vi "Write configuration.vi"(8 "error in (no error)":errorcluster, 11 "Template in":refnum<class "Cobolt.lvclass">=refnum) -> (0 "error out":errorcluster, 3 "Template out":refnum<class "Cobolt.lvclass">)   [LabVIEW 2012, in "Cobolt.lvclass"]
doc: "Writes the configuration cluster into the configuration file. Configuration file is XML-based. It's name is <component ID>.xml"
uses:
  Cobolt.lvclass
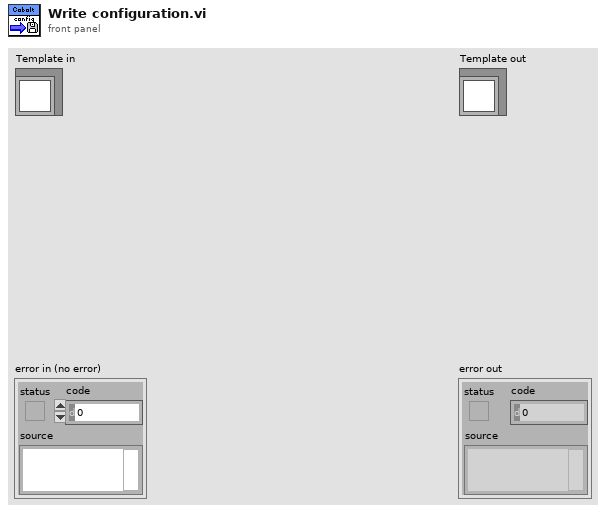
[diagram p1: front panel]
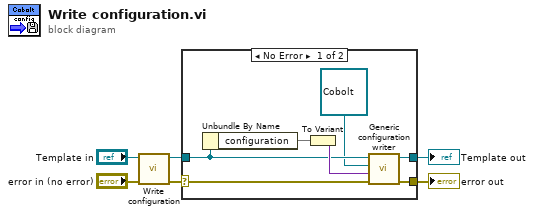
[diagram p0: block diagram]
diagram:
  n1 = call-parent "Write configuration.vi"("error in (no error)"="error in (no error)", "Murmex in"="Template in") -> ("error out"=w4:errorcluster, "Murmex out"=w2:refnum<class "Cobolt.lvclass">)  [unwired: 8 in]
  n2 = case shown="No Error" w4 {
    selector: w4 -> [w12 w15]
    tunnel: [w11 w15] -> w3
    tunnel: [w8 w14] -> w1
    tunnel: w2 -> [w9 w14]
    frame No Error {
      n3 = Unbundle By Name(w9) -> ("configuration"=w13)
      n4 = To Variant(anything=w13) -> (Variant=w10:variant)
      n5 = call "Generic configuration writer.vi"("error in (no error)"=w12, "configuration"=w10, "inheritance level"=refnum<class "Cobolt.lvclass"> refnum ("Template.lvclass"), "MurmexBase in"=w9) -> ("error out"=w11:errorcluster, "MurmexBase out"=w8:refnum<class "Cobolt.lvclass">)  [unwired: 6 in]
    }
    frame Error {
    }
  }
  "error out" <- w3
  "Template out" <- w1
